vi "一体站流程自动启动.vi"(11 "参数":T1) -> ()   [LabVIEW 2016, in "PLC.lvlib"]
uses:
  PLC.lvlib
  <vilib>/ptbypt/NI_PtbyPt.lvlib
panel:
  out "s? t:f":enum16{"初始化", "采配水启动", "仪器操作", "反冲洗", "结束"}(ring)
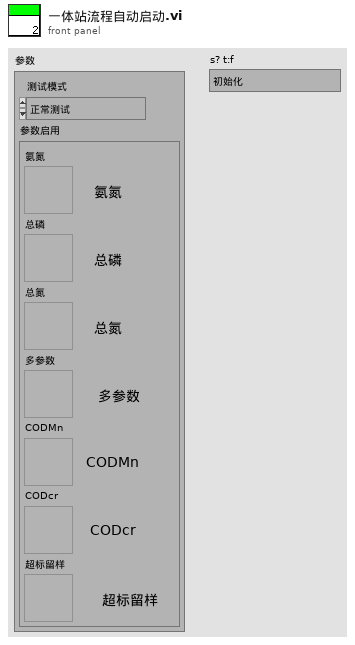
[diagram p1: front panel]
types:
  T1 = cluster{"测试模式":enum16{"正常测试", "集成干预"}, "参数启用":cluster{"氨氮":bool, "总磷":bool, "总氮":bool, "多参数":bool, "CODMn":bool, "CODcr":bool, "超标留样":bool}}
  T2 = cluster{"命令":string, cluster{"starting address":u16, "holding register value":u16}}
  T3 = enum16{"加标流程（润洗/采样分开）", "加标流程（润洗/采样合并）", "加标流程（不启动采配水）", "水样测试（润洗/采样分开）", "水样测试（润洗/采样合并）", "水样测试（不启动采配水）"}
  T4 = typedef "质控单元V4.lvlib/质控slave id.ctl" = enum16{"null", "氨氮", "总磷", "总氮", "CODMn", "CODCr", "氨氮总磷", "总磷总氮"}
  T5 = enum32{"Bad", "Idle", "Run top level", "Running"}
  T6 = cluster{"R0":i16, "R1":i16, "R2":i16, "R3":i16, "R4":i16, "R5":i16, "R6":i16, "R7":i16, "R8":i16, "R9":i16, "R10":i16, "R11":i16, "R12":i16, "R13":i16, "R14":i16, "R15":i16, "R16":i16, "R17":i16, "R18":i16, "R19":i16, "R20":i16, "R21":i16, "R22":i16, "R23":i16, "R24":i16, "R25":i16, "R26":i16, "R27":i16, "R28":i16, "R29":i16, "R30":i16, "R31":i16, "R32":i16, "R33":i16, "R34":i16, "R35":i16, "R36":i16, "R37":i16, "R38":i16, "R39":i16}
  T7 = cluster{"氨氮":bool, "总磷":bool, "总氮":bool, "多参数":bool, "CODmn":bool, "CODCr":bool, "超标留样":bool}
  T8 = cluster{"因子编码":u32, "单位":u16, "标样参考值":sgl, "水样数据时间":timestamp, "水样实测值":sgl, "水样数据标识":string, "标样数据时间":timestamp, "标样实测值":sgl, "标样数据标识":string, "空白数据时间":timestamp, "空白实测值":sgl, "空白数据标识":string, "零点核查数据时间":timestamp, "零点核查实测值":sgl, "零点核查数据标识":string, "跨度核查数据时间":timestamp, "跨度核查实测值":sgl, "跨度核查数据标识":string, "加标回收数据时间":timestamp, "加标回收实测值":sgl, "加标回收数据标识":string, "平行样数据时间":timestamp, "平行样实测值":sgl, "平行样数据标识":string, "F0":sgl, "F1":sgl, "F2":sgl, "F3":sgl, "F4":sgl, "F5":sgl, "F6":sgl, "F7":sgl, "温度":sgl, "湿度":sgl, "X值":sgl, "fidrange":u16}
  T9 = cluster{"因子编码":u32, "单位":u16, "标样参考值":sgl, "水样数据时间":timestamp, "水样实测值":sgl, "水样数据标识":string, "标样数据时间":timestamp, "标样实测值":sgl, "标样数据标识":string, "空白数据时间":timestamp, "空白实测值":sgl, "空白数据标识":string, "零点核查数据时间":timestamp, "零点核查实测值":sgl, "零点核查数据标识":string, "跨度核查数据时间":timestamp, "跨度核查实测值":sgl, "跨度核查数据标识":string, "加标回收数据时间":timestamp, "加标回收实测值":sgl, "加标回收数据标识":string, "平行样数据时间":timestamp, "平行样实测值":sgl, "平行样数据标识":string}
  T10 = cluster{"氨氮":bool, "总磷":bool, "总氮":bool, "多参数":bool, "CODMn":bool, "CODcr":bool, "超标留样":bool}
  T11 = cluster{"时间标识":timestamp, "参数":string, "数据类型":string, "集成干预测试浓度值":dbl, "集成干预前测试时间":timestamp, "集成干预前测试浓度值":dbl}
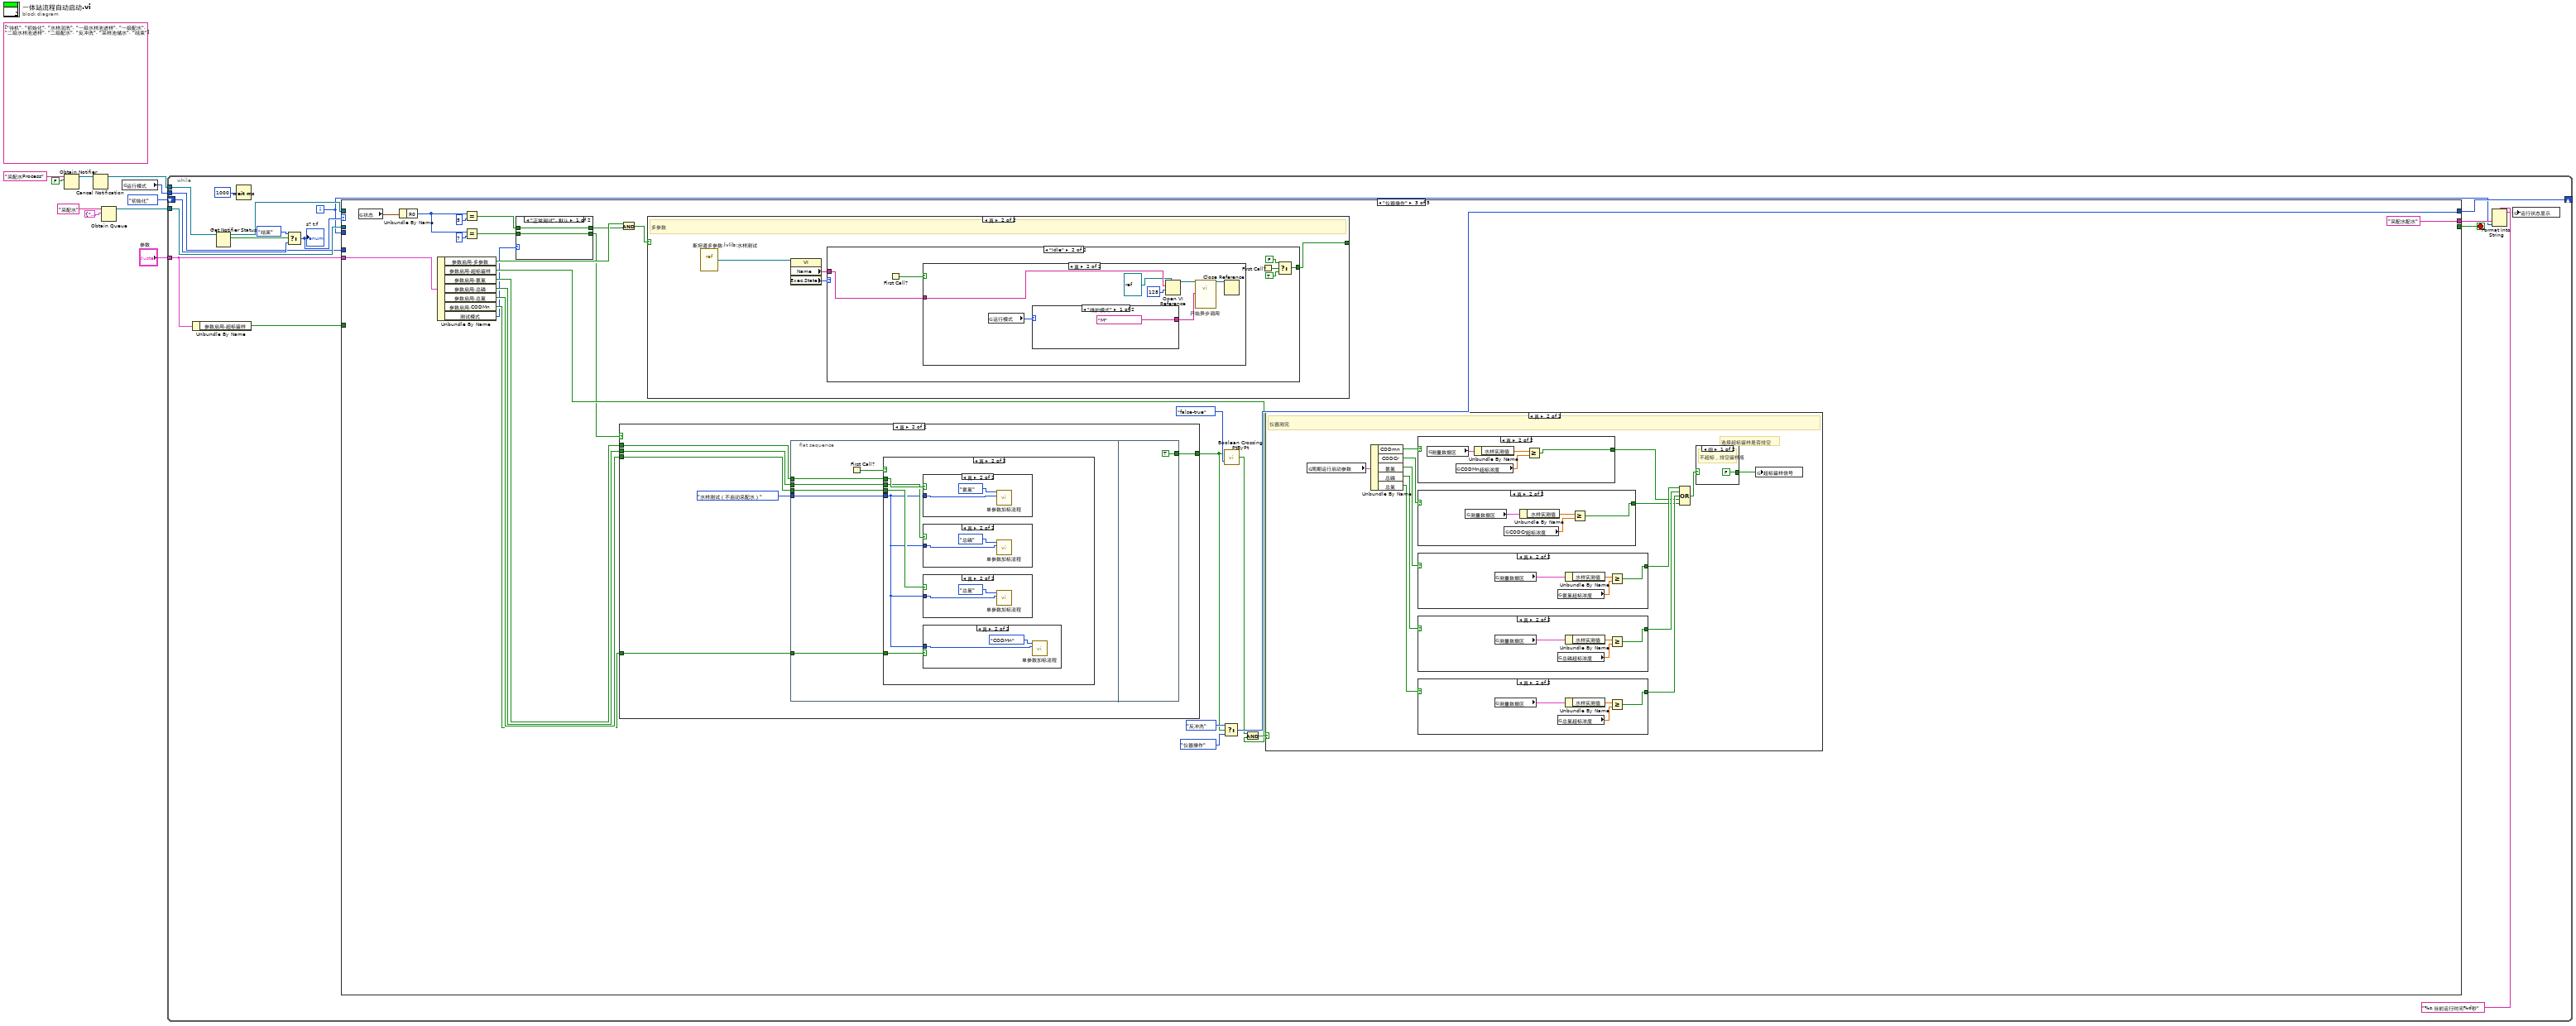
[diagram p0: block diagram]
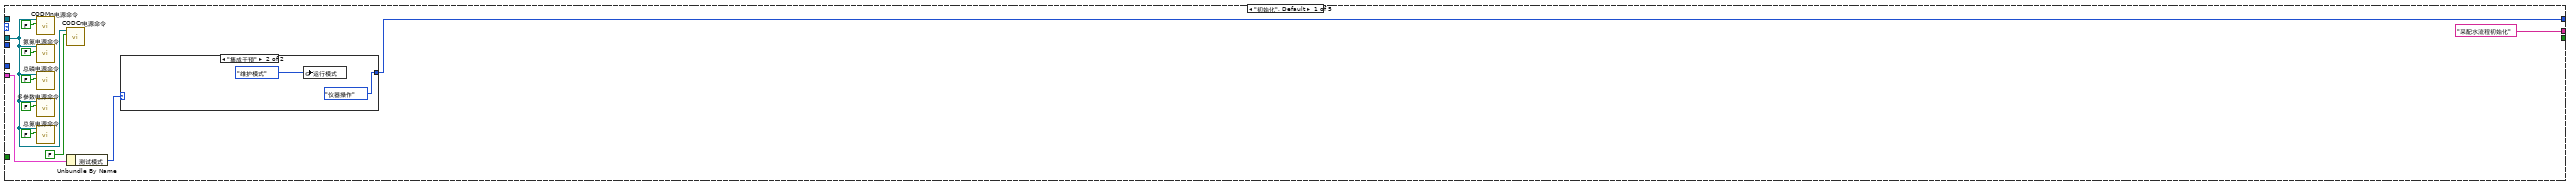
[diagram p2: hidden frame]
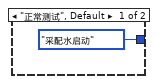
[diagram p3: hidden frame]
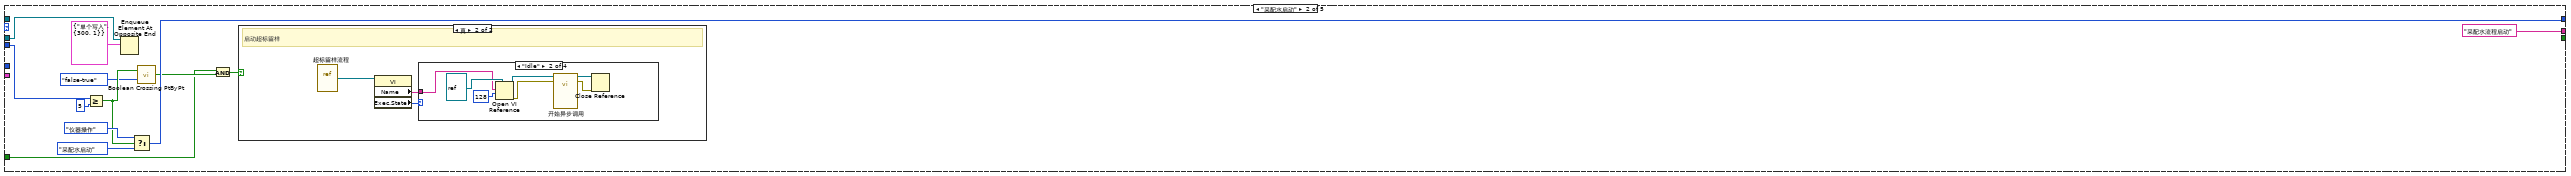
[diagram p4: hidden frame]
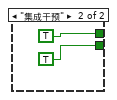
[diagram p9: hidden frame]
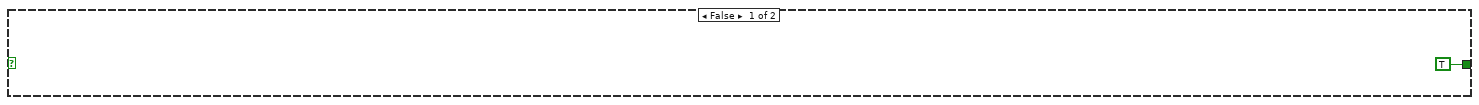
[diagram p16: hidden frame]
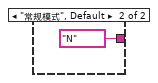
[diagram p19: hidden frame]
diagram:
  (unwired) string[][] [["待机"], ["初始化"], ["水样润洗"], ["一级水样池进样"], ["一级配水"], ["二级水样池进样"], ["二级配水"], ["反冲洗"], ["采样池储水"], ["结束"]] ("项名")
  n1 = Obtain Notifier(name (unnamed)="采配水Process" ("名称（未命名）"), notification data type=FALSE) -> (notifier out=w4:refnum<notifier>)  [unwired: 2 in, 2 out]
  n2 = Cancel Notification(0:w4) -> (8:w3:refnum<notifier>)  [unwired: 1 in, 2 out]
  n3 = Obtain Queue(name (unnamed)="采配水" ("名称（未命名）"), element data type=cluster{"命令":string, "数据":variant} {"命令"="", "数据"=variant}) -> (queue out=w7:refnum<queue>)  [unwired: 3 in, 2 out]
  n4 = global read "系统设置全局变量.vi" "运行模式"() -> (w1:enum16{"维护模式", "常规模式", "应急模式", "质控模式"})
  n5 = while {
    shift-right: [w24] -> _
    shift-left: enum16{"初始化", "采配水启动", "仪器操作", "反冲洗", "结束"}."初始化" ("枚举") -> [w20]
    tunnel: w7 -> [w27]
    tunnel: w3 -> [w23]
    tunnel: "参数" -> [w12]
    tunnel: w1 -> [w14]
    i -> [w13]
    stop <- w26 stop-if-true
    n6 = Unbundle By Name(w12) -> ("参数启用.超标留样"=w11:bool)
    n7 = Get Notifier Status(notifier=w23) -> (notifier out=w15:refnum<notifier>, current notification=w22:bool)  [unwired: 1 in, 3 out]
    n8 = Wait (ms)(milliseconds to wait=u32 1000 ("等待时间（毫秒）")) -> ()  [unwired: 1 out]
    n9 = Select(t=enum16{"初始化", "采配水启动", "仪器操作", "反冲洗", "结束"}."结束" ("枚举"), s=w22, f=w20) -> (s? t:f=w19:enum16{"初始化", "采配水启动", "仪器操作", "反冲洗", "结束"})
    "s? t:f" <- w19
    n10 = case shown="\"仪器操作\"" w19 {
      tunnel: w27 -> [w29 w54 _ _ w381]
      tunnel: [_ _ _ _ TRUE] -> w26
      tunnel: [w33 w48 w86 w184 enum16{"初始化", "采配水启动", "仪器操作", "反冲洗", "结束"}."结束" ("枚举")] -> w24
      tunnel: ["采配水流程初始化" "采配水流程启动" "采配水配水" "等待测试完成" "采配水结束"] -> w16
      tunnel: w15 -> [_ _ _ _ w382]
      tunnel: w12 -> [w31 _ w88 w183 w378]
      tunnel: w14 -> [_ _ _ w180 w377]
      tunnel: w13 -> [_ w52 _ _ _]
      tunnel: w11 -> [_ w43 _ _ _]
      frame "初始化", Default {
        n11 = call "CODMn电源命令.vi"("通电/断电"=FALSE, "队列"=w29) -> ()  [unwired: 9 in, 1 out]
        n12 = call "氨氮电源命令.vi"("通电/断电"=FALSE, "队列"=w29) -> ()  [unwired: 9 in, 1 out]
        n13 = call "总磷电源命令.vi"("通电/断电"=FALSE, "队列"=w29) -> ()  [unwired: 9 in, 1 out]
        n14 = call "多参数电源命令.vi"("通电/断电"=FALSE, "队列"=w29) -> ()  [unwired: 9 in, 1 out]
        n15 = call "总氮电源命令.vi"("通电/断电"=FALSE, "队列"=w29) -> ()  [unwired: 9 in, 1 out]
        n16 = call "CODCr电源命令.vi"("通电/断电"=FALSE, "队列"=w29) -> ()  [unwired: 9 in, 1 out]
        n17 = Unbundle By Name(w31) -> ("测试模式"=w30:enum16{"正常测试", "集成干预"})
        n18 = case shown="\"集成干预\"" w30 {
          tunnel: [enum16{"初始化", "采配水启动", "仪器操作", "反冲洗", "结束"}."采配水启动" ("枚举") enum16{"初始化", "采配水启动", "仪器操作", "反冲洗", "结束"}."仪器操作" ("枚举")] -> w33
          frame "正常测试", Default {
          }
          frame "集成干预" {
            n19 = global write "系统设置全局变量.vi" "运行模式"(enum16{"维护模式", "常规模式", "应急模式", "质控模式"}."维护模式" ("运行模式")) -> ()
          }
        }
      }
      frame "采配水启动" {
        n20 = Greater Or Equal?(x=w52, y=5) -> (x >= y?=w47:bool)
        n21 = Enqueue Element At Opposite End(queue=w54, element=T2 {"命令"="单个写入", {"starting address"=300, "holding register value"=1}} ("元素")) -> ()  [unwired: 2 in, 3 out]
        n22 = Select(t=enum16{"初始化", "采配水启动", "仪器操作", "反冲洗", "结束"}."仪器操作" ("枚举"), s=w47, f=enum16{"初始化", "采配水启动", "仪器操作", "反冲洗", "结束"}."采配水启动" ("枚举")) -> (s? t:f=w48:enum16{"初始化", "采配水启动", "仪器操作", "反冲洗", "结束"})
        n23 = call <vilib>:"Boolean Crossing PtByPt.vi"("direction"=enum16{"either", "false-true", "true-false"}."false-true", "input"=w47) -> ("crossing"=w45:bool)  [unwired: 1 in]
        n24 = And(x=w43, y=w45) -> (x .and. y?=w44:bool)
        n25 = case shown="真" w44 {
          frame False {
          }
          frame True {
            # "启动超标留样"
            n26 = vi-ref "超标留样流程.vi"() -> (w57:refnum<vi>)
            n27 = property class="VI"(reference=w57) -> ("Name"=w56:string, "Exec.State"=w55:T5)  [unwired: 1 in, 2 out]
            n28 = case shown="\"Idle\"" w55 {
              tunnel: w56 -> [_ w60 _ _]
              frame "Bad", Default {
              }
              frame "Idle" {
                n29 = Open VI Reference(type specifier VI Refnum (for type only)=refnum<vi> refnum ("类型说明符VI引用句柄（仅用于类型）"), vi path=w60, options=128 ("选项")) -> (vi reference=w64:refnum<vi>, error out=w59:errorcluster)  [unwired: 3 in]
                n30 = call-by-ref "开始异步调用"(reference=w64, error in=w59) -> (reference out=w63:refnum<vi>, error out=w58:errorcluster)  [unwired: 12 in]
                n31 = Close Reference(reference=w63, error in (no error)=w58) -> ()  [unwired: 1 out]
              }
              frame "Run top level" {
              }
              frame "Running" {
              }
            }
          }
        }
      }
      frame "仪器操作" {
        n32 = global read "采配水全局变量.vi" "状态"() -> (w75:T6)
        n33 = Unbundle By Name(w75) -> ("R0"=w71:i16)
        n34 = Unbundle By Name(w88) -> ("参数启用.多参数"=w81:bool, "参数启用.超标留样"=w82:bool, "参数启用.氨氮"=w79:bool, "参数启用.总磷"=w78:bool, "参数启用.总氮"=w77:bool, "参数启用.CODMn"=w76:bool, "测试模式"=w69:enum16{"正常测试", "集成干预"})
        n35 = Equal?(x=w71, y=i16 5) -> (x = y?=w68:bool)
        n36 = Equal?(x=w71, y=i16 7) -> (x = y?=w66:bool)
        n37 = case shown="\"正常测试\", 默认" w69 {
          tunnel: w68 -> [w91 _]
          tunnel: [w91 TRUE] -> w67
          tunnel: w66 -> [w90 _]
          tunnel: [w90 TRUE] -> w65
          frame "正常测试", Default {
          }
          frame "集成干预" {
          }
        }
        n38 = case shown="真" w65 {
          tunnel: [_ w98] -> w80
          tunnel: w79 -> [_ w97]
          tunnel: w78 -> [_ w96]
          tunnel: w77 -> [_ w95]
          tunnel: w76 -> [_ w94]
          frame False {
          }
          frame True {
            n39 = flat-sequence {
              tunnel: T3."水样测试（不启动采配水）" ("流程类型") -> [w101]
              tunnel: w97 -> [w105]
              tunnel: w96 -> [w104]
              tunnel: w95 -> [w103]
              tunnel: w94 -> [w102]
              tunnel: [TRUE] -> w98
              frame #0 {
                n40 = First Call?() -> (First Call?: T/F=w100:bool)
                n41 = case shown="真" w100 {
                  tunnel: w105 -> [_ w110]
                  tunnel: w104 -> [_ w109]
                  tunnel: w103 -> [_ w108]
                  tunnel: w102 -> [_ w107]
                  tunnel: w101 -> [_ w106]
                  frame False {
                  }
                  frame True {
                    n42 = case shown="真" w110 {
                      tunnel: w106 -> [_ w117]
                      frame False {
                      }
                      frame True {
                        n43 = call "单参数加标流程.vi"("流程类型"=w117, "Slave ID"=质控slave_id."氨氮") -> ()  [unwired: 10 in]
                      }
                    }
                    n44 = case shown="真" w109 {
                      tunnel: w106 -> [_ w115]
                      frame False {
                      }
                      frame True {
                        n45 = call "单参数加标流程.vi"("流程类型"=w115, "Slave ID"=质控slave_id."总磷") -> ()  [unwired: 10 in]
                      }
                    }
                    n46 = case shown="真" w108 {
                      tunnel: w106 -> [_ w113]
                      frame False {
                      }
                      frame True {
                        n47 = call "单参数加标流程.vi"("流程类型"=w113, "Slave ID"=质控slave_id."总氮") -> ()  [unwired: 10 in]
                      }
                    }
                    n48 = case shown="真" w107 {
                      tunnel: w106 -> [_ w111]
                      frame False {
                      }
                      frame True {
                        n49 = call "单参数加标流程.vi"("流程类型"=w111, "Slave ID"=质控slave_id."CODMn") -> ()  [unwired: 10 in]
                      }
                    }
                  }
                }
              }
              frame #1 {
              }
            }
          }
        }
        n50 = And(x=w81, y=w67) -> (x .and. y?=w73:bool)
        n51 = case shown="真" w73 {
          tunnel: [TRUE ("t") w124] -> _
          frame False {
          }
          frame True {
            # "多参数"
            n52 = vi-ref "斯坦道多参数.lvlib:水样测试.vi"() -> (w122:refnum<vi>)
            n53 = property class="VI"(reference=w122) -> ("Name"=w121:string, "Exec.State"=w123:T5)  [unwired: 1 in, 2 out]
            n54 = case shown="\"Idle\"" w123 {
              tunnel: w121 -> [_ w130]
              tunnel: [_ w125] -> w124
              frame "Bad", Default {
              }
              frame "Idle" {
                n55 = First Call?() -> (First Call?: T/F=w129:bool)
                n56 = case shown="真" w129 {
                  tunnel: w130 -> [_ w136]
                  frame False {
                  }
                  frame True {
                    n57 = global read "系统设置全局变量.vi" "运行模式"() -> (w133:enum16{"维护模式", "常规模式", "应急模式", "质控模式"})
                    n58 = case shown="\"维护模式\"" w133 {
                      tunnel: ["M" ("数据标记表") "N" ("数据标记表")] -> w132
                      frame "维护模式" {
                      }
                      frame "常规模式", Default {
                      }
                    }
                    n59 = Open VI Reference(type specifier VI Refnum (for type only)=refnum<vi> refnum, vi path=w136, options=128 ("选项")) -> (vi reference=w135:refnum<vi>)  [unwired: 3 in, 1 out]
                    n60 = call-by-ref "开始异步调用"(reference=w135, "数据标记表"=w132) -> (reference out=w134:refnum<vi>)  [unwired: 12 in, 1 out]
                    n61 = Close Reference(reference=w134) -> ()  [unwired: 1 in, 1 out]
                  }
                }
                n62 = First Call?() -> (First Call?: T/F=w128:bool)
                n63 = Select(t=FALSE, s=w128, f=TRUE) -> (s? t:f=w125:bool)
              }
            }
          }
        }
        n64 = Select(t=enum16{"初始化", "采配水启动", "仪器操作", "反冲洗", "结束"}."反冲洗" ("枚举"), s=w80, f=enum16{"初始化", "采配水启动", "仪器操作", "反冲洗", "结束"}."仪器操作" ("枚举")) -> (s? t:f=w86:enum16{"初始化", "采配水启动", "仪器操作", "反冲洗", "结束"})
        n65 = call <vilib>:"Boolean Crossing PtByPt.vi"("direction"=enum16{"either", "false-true", "true-false"}."false-true", "input"=w80) -> ("crossing"=w84:bool)  [unwired: 1 in]
        n66 = And(x=w84, y=w82) -> (x .and. y?=w83:bool)
        n67 = case shown="真" w83 {
          frame False {
          }
          frame True {
            # "选择超标留样是否排空"
            # "仪器测完"
            n68 = global read "系统设置全局变量.vi" "周期运行启动参数"() -> (w146:T7)
            n69 = Unbundle By Name(w146) -> ("CODmn"=w145:bool, "CODCr"=w144:bool, "氨氮"=w143:bool, "总磷"=w142:bool, "总氮"=w141:bool)
            n70 = case shown="真" w145 {
              tunnel: [FALSE w164] -> w149
              frame False {
              }
              frame True {
                n71 = global read "VARCODMn全局变量.vi" "测量数据区"() -> (w162:T8)
                n72 = global read "外部交互全局.vi" "CODMn超标浓度"() -> (w163:dbl)
                n73 = Unbundle By Name(w162) -> ("水样实测值"=w161:sgl)
                n74 = Greater Or Equal?(x=w161, y=w163) -> (x >= y?=w164:bool)
              }
            }
            n75 = case shown="真" w144 {
              tunnel: [FALSE w157] -> w148
              frame False {
              }
              frame True {
                n76 = global read "CODcr全局变量.vi" "测量数据区"() -> (w159:T9)
                n77 = global read "外部交互全局.vi" "CODCr超标浓度"() -> (w156:dbl)
                n78 = Unbundle By Name(w159) -> ("水样实测值"=w158:sgl)
                n79 = Greater Or Equal?(x=w158, y=w156) -> (x >= y?=w157:bool)
              }
            }
            n80 = case shown="真" w143 {
              tunnel: [FALSE w177] -> w152
              frame False {
              }
              frame True {
                n81 = global read "VAR总磷总氮全局变量.vi" "测量数据区"() -> (w179:T8)
                n82 = global read "外部交互全局.vi" "氨氮超标浓度"() -> (w176:dbl)
                n83 = Unbundle By Name(w179) -> ("水样实测值"=w178:sgl)
                n84 = Greater Or Equal?(x=w178, y=w176) -> (x >= y?=w177:bool)
              }
            }
            n85 = case shown="真" w142 {
              tunnel: [FALSE w172] -> w151
              frame False {
              }
              frame True {
                n86 = global read "VAR总磷总氮全局变量.vi" "测量数据区"() -> (w174:T8)
                n87 = global read "外部交互全局.vi" "总磷超标浓度"() -> (w171:dbl)
                n88 = Unbundle By Name(w174) -> ("水样实测值"=w173:sgl)
                n89 = Greater Or Equal?(x=w173, y=w171) -> (x >= y?=w172:bool)
              }
            }
            n90 = case shown="真" w141 {
              tunnel: [FALSE w167] -> w150
              frame False {
              }
              frame True {
                n91 = global read "VAR总磷总氮全局变量.vi" "测量数据区"() -> (w169:T8)
                n92 = global read "外部交互全局.vi" "总氮超标浓度"() -> (w166:dbl)
                n93 = Unbundle By Name(w169) -> ("水样实测值"=w168:sgl)
                n94 = Greater Or Equal?(x=w168, y=w166) -> (x >= y?=w167:bool)
              }
            }
            n95 = Compound Arithmetic op=OR ("复合运算")(w152, w151, w150, w149, w148) -> (w147:bool)
            n96 = case shown="假" w147 {
              tunnel: [FALSE ("超标留样信号") TRUE ("超标留样信号")] -> w140
              frame False {
                # "不超标，排空留样瓶"
              }
              frame True {
                # "超标"
              }
            }
            n97 = global write "外部交互全局.vi" "超标留样信号"(w140) -> ()
          }
        }
      }
      frame "反冲洗" {
        n98 = First Call?() -> (First Call?: T/F=w181:bool)
        n99 = case shown="真" w181 {
          tunnel: w183 -> [_ w193]
          tunnel: w180 -> [_ w190]
          frame False {
          }
          frame True {
            n100 = Unbundle By Name(w193) -> ("测试模式"=w192:enum16{"正常测试", "集成干预"}, "参数启用"=w191:T10)
            n101 = case shown="\"正常测试\", 默认" w192 {
              tunnel: w191 -> [w196 w302]
              tunnel: w190 -> [_ w290]
              frame "正常测试", Default {
                n102 = global read "系统设置全局变量.vi" "运行模式"() -> (w194:enum16{"维护模式", "常规模式", "应急模式", "质控模式"})
                n103 = global read "采配水全局变量.vi" "报警簇"() -> (w201:bool[])
                n104 = case shown="\"常规模式\", 默认" w194 {
                  tunnel: ["M" ("table") "N" ("table")] -> w195
                  frame "维护模式" {
                  }
                  frame "常规模式", Default {
                  }
                }
                n105 = Index Array(array=w201, index #1=0 ("索引"), index #2=11 ("索引")) -> (element #1=w198:bool, element #2=w197:bool)
                n106 = case shown="真" w198 {
                  tunnel: w197 -> [w207 _]
                  tunnel: w196 -> [w206 w227]
                  tunnel: w195 -> [w204 w215]
                  frame False {
                    n107 = Unbundle By Name(w206) -> ("氨氮"=w205:bool)
                    n108 = case shown="真" w207 {
                      tunnel: w205 -> [_ w209]
                      tunnel: w204 -> [_ w208]
                      frame False {
                      }
                      frame True {
                        n109 = case shown="真" w209 {
                          tunnel: w208 -> [_ w210]
                          tunnel: [_ w211] -> _
                          frame False {
                          }
                          frame True {
                            n110 = call "取水点无水样数据存储.vi"("数据标识"="lw", "数据类型"=w210, "table"="氨氮") -> ("error out"=w211:errorcluster)  [unwired: 8 in]
                          }
                        }
                      }
                    }
                  }
                  frame True {
                    n111 = global read "采配水全局变量.vi" "输入状态"() -> (w220:bool[])
                    n112 = Index Array(array=w220, index=4 ("索引")) -> (element=w218:bool)
                    n113 = Unbundle By Name(w227) -> ("氨氮"=w226:bool, "CODMn"=w225:bool, "CODcr"=w224:bool, "多参数"=w223:bool, "总氮"=w222:bool, "总磷"=w221:bool)
                    n114 = Select(t="P" ("数据标识"), s=w218, f="Z" ("数据标识")) -> (s? t:f=w214:string)
                    n115 = case shown="真" w223 {
                      tunnel: w215 -> [_ w249]
                      tunnel: w214 -> [_ w241]
                      tunnel: w214 -> [_ w240]
                      tunnel: w214 -> [_ w239]
                      tunnel: w214 -> [_ w238]
                      tunnel: w214 -> [_ w237]
                      tunnel: w214 -> [_ w236]
                      tunnel: w214 -> [_ w235]
                      frame False {
                      }
                      frame True {
                        n116 = global read "断电保存变量.vi" "Cond"() -> (w244:bool)
                        n117 = global read "断电保存变量.vi" "Turb"() -> (w245:bool)
                        n118 = global read "断电保存变量.vi" "DO"() -> (w246:bool)
                        n119 = global read "断电保存变量.vi" "pH"() -> (w247:bool)
                        n120 = global read "断电保存变量.vi" "藻密度"() -> (w242:bool)
                        n121 = global read "断电保存变量.vi" "Temp"() -> (w248:bool)
                        n122 = case shown="真" w247 {
                          tunnel: w249 -> [_ w272]
                          tunnel: [_ w271] -> _
                          tunnel: w241 -> [_ w270]
                          frame False {
                          }
                          frame True {
                            n123 = call "取水点无水样数据存储.vi"("数据标识"=w270, "数据类型"=w272, "table"="pH") -> ("error out"=w271:errorcluster)  [unwired: 8 in]
                          }
                        }
                        n124 = case shown="真" w246 {
                          tunnel: w249 -> [_ w268]
                          tunnel: [_ w267] -> _
                          tunnel: w240 -> [_ w266]
                          frame False {
                          }
                          frame True {
                            n125 = call "取水点无水样数据存储.vi"("数据标识"=w266, "数据类型"=w268, "table"="DO") -> ("error out"=w267:errorcluster)  [unwired: 8 in]
                          }
                        }
                        n126 = case shown="真" w245 {
                          tunnel: w249 -> [_ w260]
                          tunnel: [_ w259] -> _
                          tunnel: w239 -> [_ w258]
                          frame False {
                          }
                          frame True {
                            n127 = call "取水点无水样数据存储.vi"("数据标识"=w258, "数据类型"=w260, "table"="浊度") -> ("error out"=w259:errorcluster)  [unwired: 8 in]
                          }
                        }
                        n128 = case shown="真" w244 {
                          tunnel: w249 -> [_ w264]
                          tunnel: [_ w263] -> _
                          tunnel: w237 -> [_ w262]
                          frame False {
                          }
                          frame True {
                            n129 = call "取水点无水样数据存储.vi"("数据标识"=w262, "数据类型"=w264, "table"="比电导率") -> ("error out"=w263:errorcluster)  [unwired: 8 in]
                          }
                        }
                        n130 = global read "断电保存变量.vi" "叶绿素a启用"() -> (w243:bool)
                        n131 = case shown="真" w248 {
                          tunnel: w249 -> [_ w276]
                          tunnel: [_ w275] -> _
                          tunnel: w238 -> [_ w274]
                          frame False {
                          }
                          frame True {
                            n132 = call "取水点无水样数据存储.vi"("数据标识"=w274, "数据类型"=w276, "table"="水温") -> ("error out"=w275:errorcluster)  [unwired: 8 in]
                          }
                        }
                        n133 = case shown="真" w242 {
                          tunnel: w249 -> [_ w252]
                          tunnel: [_ w251] -> _
                          tunnel: w236 -> [_ w250]
                          frame False {
                          }
                          frame True {
                            n134 = call "取水点无水样数据存储.vi"("数据标识"=w250, "数据类型"=w252, "table"="藻密度") -> ("error out"=w251:errorcluster)  [unwired: 8 in]
                          }
                        }
                        n135 = case shown="真" w243 {
                          tunnel: w249 -> [_ w256]
                          tunnel: [_ w255] -> _
                          tunnel: w235 -> [_ w254]
                          frame False {
                          }
                          frame True {
                            n136 = call "取水点无水样数据存储.vi"("数据标识"=w254, "数据类型"=w256, "table"="叶绿素a") -> ("error out"=w255:errorcluster)  [unwired: 8 in]
                          }
                        }
                      }
                    }
                    n137 = case shown="真" w226 {
                      tunnel: w215 -> [_ w287]
                      tunnel: [_ w288] -> _
                      tunnel: w214 -> [_ w286]
                      frame False {
                      }
                      frame True {
                        n138 = call "取水点无水样数据存储.vi"("数据标识"=w286, "数据类型"=w287, "table"="氨氮") -> ("error out"=w288:errorcluster)  [unwired: 8 in]
                      }
                    }
                    n139 = case shown="真" w222 {
                      tunnel: w215 -> [_ w233]
                      tunnel: w214 -> [_ w232]
                      frame False {
                      }
                      frame True {
                        n140 = call "取水点无水样数据存储.vi"("数据标识"=w232, "数据类型"=w233, "table"="总氮") -> ()  [unwired: 8 in, 1 out]
                      }
                    }
                    n141 = case shown="真" w221 {
                      tunnel: [_ w230] -> _
                      tunnel: w214 -> [_ w229]
                      tunnel: w215 -> [_ w228]
                      frame False {
                      }
                      frame True {
                        n142 = call "取水点无水样数据存储.vi"("数据标识"=w229, "数据类型"=w228, "table"="总磷") -> ("error out"=w230:errorcluster)  [unwired: 8 in]
                      }
                    }
                    n143 = case shown="真" w225 {
                      tunnel: w215 -> [_ w284]
                      tunnel: [_ w283] -> _
                      tunnel: w214 -> [_ w282]
                      frame False {
                      }
                      frame True {
                        n144 = call "取水点无水样数据存储.vi"("数据标识"=w282, "数据类型"=w284, "table"="CODMn") -> ("error out"=w283:errorcluster)  [unwired: 8 in]
                      }
                    }
                    n145 = case shown="真" w224 {
                      tunnel: w215 -> [_ w280]
                      tunnel: [_ w279] -> _
                      tunnel: w214 -> [_ w278]
                      frame False {
                      }
                      frame True {
                        n146 = call "取水点无水样数据存储.vi"("数据标识"=w278, "数据类型"=w280, "table"="CODCr") -> ("error out"=w279:errorcluster)  [unwired: 8 in]
                      }
                    }
                  }
                }
              }
              frame "集成干预" {
                n147 = Unbundle By Name(w302) -> ("总磷"=w296:bool, "总氮"=w297:bool, "氨氮"=w301:bool, "CODMn"=w300:bool, "CODcr"=w299:bool, "多参数"=w298:bool)
                n148 = case shown="真" w296 {
                  tunnel: [_ w309] -> w295
                  tunnel: w290 -> [_ w308]
                  frame False {
                  }
                  frame True {
                    n149 = call "获取最近两组水样测试数据.vi"("运行模式"=w308, "table"="总磷") -> ("error out"=w312:errorcluster, "存储变量"=w311:T11)  [unwired: 8 in]
                    n150 = call "集成干预测试数据存储.vi"("error in (no error)"=w312, "存储变量"=w311) -> ("error out"=w309:errorcluster)  [unwired: 9 in]
                  }
                }
                n151 = case shown="真" w297 {
                  tunnel: w295 -> [_ _]
                  tunnel: [_ w304] -> w294
                  tunnel: w290 -> [_ w303]
                  frame False {
                  }
                  frame True {
                    n152 = call "获取最近两组水样测试数据.vi"("运行模式"=w303, "table"="总氮") -> ("error out"=w307:errorcluster, "存储变量"=w306:T11)  [unwired: 8 in]
                    n153 = call "集成干预测试数据存储.vi"("error in (no error)"=w307, "存储变量"=w306) -> ("error out"=w304:errorcluster)  [unwired: 9 in]
                  }
                }
                n154 = case shown="真" w301 {
                  tunnel: w294 -> [_ _]
                  tunnel: [_ w373] -> w291
                  tunnel: w290 -> [_ w372]
                  frame False {
                  }
                  frame True {
                    n155 = call "获取最近两组水样测试数据.vi"("运行模式"=w372, "table"="氨氮") -> ("error out"=w374:errorcluster, "存储变量"=w375:T11)  [unwired: 8 in]
                    n156 = call "集成干预测试数据存储.vi"("error in (no error)"=w374, "存储变量"=w375) -> ("error out"=w373:errorcluster)  [unwired: 9 in]
                  }
                }
                n157 = case shown="真" w300 {
                  tunnel: [_ w368] -> w293
                  tunnel: w291 -> [_ _]
                  tunnel: w290 -> [_ w367]
                  frame False {
                  }
                  frame True {
                    n158 = call "获取最近两组水样测试数据.vi"("运行模式"=w367, "table"="CODMn") -> ("error out"=w369:errorcluster, "存储变量"=w370:T11)  [unwired: 8 in]
                    n159 = call "集成干预测试数据存储.vi"("error in (no error)"=w369, "存储变量"=w370) -> ("error out"=w368:errorcluster)  [unwired: 9 in]
                  }
                }
                n160 = case shown="真" w299 {
                  tunnel: w293 -> [_ _]
                  tunnel: [_ w363] -> w292
                  frame False {
                  }
                  frame True {
                    n161 = global read "系统设置全局变量.vi" "运行模式"() -> (w362:enum16{"维护模式", "常规模式", "应急模式", "质控模式"})
                    n162 = call "获取最近两组水样测试数据.vi"("运行模式"=w362, "table"="CODCr") -> ("error out"=w364:errorcluster, "存储变量"=w365:T11)  [unwired: 8 in]
                    n163 = call "集成干预测试数据存储.vi"("error in (no error)"=w364, "存储变量"=w365) -> ("error out"=w363:errorcluster)  [unwired: 9 in]
                  }
                }
                n164 = case shown="真" w298 {
                  tunnel: w292 -> [_ _]
                  tunnel: w290 -> [_ w313]
                  frame False {
                  }
                  frame True {
                    n165 = global read "断电保存变量.vi" "Temp"() -> (w320:bool)
                    n166 = case shown="真" w320 {
                      tunnel: [_ w358] -> w326
                      tunnel: w313 -> [_ w357]
                      frame False {
                      }
                      frame True {
                        n167 = call "获取最近两组水样测试数据.vi"("运行模式"=w357, "table"="水温") -> ("error out"=w361:errorcluster, "存储变量"=w360:T11)  [unwired: 8 in]
                        n168 = call "集成干预测试数据存储.vi"("error in (no error)"=w361, "存储变量"=w360) -> ("error out"=w358:errorcluster)  [unwired: 9 in]
                      }
                    }
                    n169 = global read "断电保存变量.vi" "pH"() -> (w319:bool)
                    n170 = case shown="真" w319 {
                      tunnel: [_ w353] -> w325
                      tunnel: w326 -> [_ _]
                      tunnel: w313 -> [_ w352]
                      frame False {
                      }
                      frame True {
                        n171 = call "获取最近两组水样测试数据.vi"("运行模式"=w352, "table"="pH") -> ("error out"=w356:errorcluster, "存储变量"=w355:T11)  [unwired: 8 in]
                        n172 = call "集成干预测试数据存储.vi"("error in (no error)"=w356, "存储变量"=w355) -> ("error out"=w353:errorcluster)  [unwired: 9 in]
                      }
                    }
                    n173 = global read "断电保存变量.vi" "DO"() -> (w318:bool)
                    n174 = case shown="真" w318 {
                      tunnel: [_ w348] -> w324
                      tunnel: w325 -> [_ _]
                      tunnel: w313 -> [_ w347]
                      frame False {
                      }
                      frame True {
                        n175 = call "获取最近两组水样测试数据.vi"("运行模式"=w347, "table"="DO") -> ("error out"=w351:errorcluster, "存储变量"=w350:T11)  [unwired: 8 in]
                        n176 = call "集成干预测试数据存储.vi"("error in (no error)"=w351, "存储变量"=w350) -> ("error out"=w348:errorcluster)  [unwired: 9 in]
                      }
                    }
                    n177 = global read "断电保存变量.vi" "Cond"() -> (w317:bool)
                    n178 = case shown="真" w317 {
                      tunnel: [_ w343] -> w323
                      tunnel: w324 -> [_ _]
                      tunnel: w313 -> [_ w342]
                      frame False {
                      }
                      frame True {
                        n179 = call "获取最近两组水样测试数据.vi"("运行模式"=w342, "table"="电导率") -> ("error out"=w346:errorcluster, "存储变量"=w345:T11)  [unwired: 8 in]
                        n180 = call "集成干预测试数据存储.vi"("error in (no error)"=w346, "存储变量"=w345) -> ("error out"=w343:errorcluster)  [unwired: 9 in]
                      }
                    }
                    n181 = global read "断电保存变量.vi" "Turb"() -> (w316:bool)
                    n182 = case shown="真" w316 {
                      tunnel: [_ w338] -> w322
                      tunnel: w323 -> [_ _]
                      tunnel: w313 -> [_ w337]
                      frame False {
                      }
                      frame True {
                        n183 = call "获取最近两组水样测试数据.vi"("运行模式"=w337, "table"="浊度") -> ("error out"=w341:errorcluster, "存储变量"=w340:T11)  [unwired: 8 in]
                        n184 = call "集成干预测试数据存储.vi"("error in (no error)"=w341, "存储变量"=w340) -> ("error out"=w338:errorcluster)  [unwired: 9 in]
                      }
                    }
                    n185 = global read "断电保存变量.vi" "叶绿素a启用"() -> (w315:bool)
                    n186 = case shown="真" w315 {
                      tunnel: [_ w333] -> w321
                      tunnel: w322 -> [_ _]
                      tunnel: w313 -> [_ w332]
                      frame False {
                      }
                      frame True {
                        n187 = call "获取最近两组水样测试数据.vi"("运行模式"=w332, "table"="叶绿素a") -> ("error out"=w336:errorcluster, "存储变量"=w335:T11)  [unwired: 8 in]
                        n188 = call "集成干预测试数据存储.vi"("error in (no error)"=w336, "存储变量"=w335) -> ("error out"=w333:errorcluster)  [unwired: 9 in]
                      }
                    }
                    n189 = global read "断电保存变量.vi" "藻密度"() -> (w314:bool)
                    n190 = case shown="真" w314 {
                      tunnel: [_ w328] -> _
                      tunnel: w321 -> [_ _]
                      tunnel: w313 -> [_ w327]
                      frame False {
                      }
                      frame True {
                        n191 = call "获取最近两组水样测试数据.vi"("运行模式"=w327, "table"="藻密度") -> ("error out"=w331:errorcluster, "存储变量"=w330:T11)  [unwired: 8 in]
                        n192 = call "集成干预测试数据存储.vi"("error in (no error)"=w331, "存储变量"=w330) -> ("error out"=w328:errorcluster)  [unwired: 9 in]
                      }
                    }
                  }
                }
              }
            }
          }
        }
        n193 = global read "采配水全局变量.vi" "状态"() -> (w189:T6)
        n194 = Unbundle By Name(w189) -> ("R0"=w188:i16)
        n195 = Equal To 0?(x=w188) -> (x = 0?=w187:bool)
        n196 = Select(t=enum16{"初始化", "采配水启动", "仪器操作", "反冲洗", "结束"}."结束" ("枚举"), s=w187, f=enum16{"初始化", "采配水启动", "仪器操作", "反冲洗", "结束"}."反冲洗" ("枚举")) -> (s? t:f=w184:enum16{"初始化", "采配水启动", "仪器操作", "反冲洗", "结束"})
      }
      frame "结束" {
        n197 = Release Queue(queue=w381) -> ()  [unwired: 2 in, 3 out]
        n198 = Unbundle By Name(w378) -> ("测试模式"=w379:enum16{"正常测试", "集成干预"})
        n199 = Cancel Notification(0:w382) -> (8:w383:refnum<notifier>)  [unwired: 1 in, 2 out]
        n200 = Release Notifier(notifier=w383) -> ()  [unwired: 2 in, 3 out]
        n201 = case shown="\"集成干预\"" w379 {
          tunnel: w377 -> [_ w386]
          frame "正常测试", Default {
          }
          frame "集成干预" {
            n202 = global write "系统设置全局变量.vi" "运行模式"(w386) -> ()
          }
        }
      }
    }
    n203 = Format Into String(format string="%s,当前运行时间%d秒" ("格式字符串"), w16, w13) -> (resulting string=w17:string)  [unwired: 2 in, 1 out]
    n204 = global write "采配水全局变量.vi" "运行状态显示"(w17) -> ()
  }
